vi "AutoTask Controller.vi"(8 "error in":errorcluster) -> ()   [LabVIEW 2015]
doc: "This VI executes continuously carrying out the current operation and responding to updates or new operations. It will often contain the timing or control code that is difficult to place directly in TeleOp. This VI generally opens all sensors and motors and isolates the rest of the robot code from knowing how the operations are carried out."
uses:
  AutoTask Setpoints.ctl
  AutoTask Operations.ctl
  <vilib>/Rock Robotics/Network Tables/NT Read Number.vi
  <vilib>/Rock Robotics/Network Tables/NT Write String.vi
  NavX/navX Library v2/navX Library v2.lvlib
  <vilib>/Rock Robotics/Network Tables/NT Write Boolean.vi
panel:
  out "Current\nCmd":string
  # "Tip: It may be helpful to observe inputs and sensor values.\nYou may also want to display tuning or debugging controls."
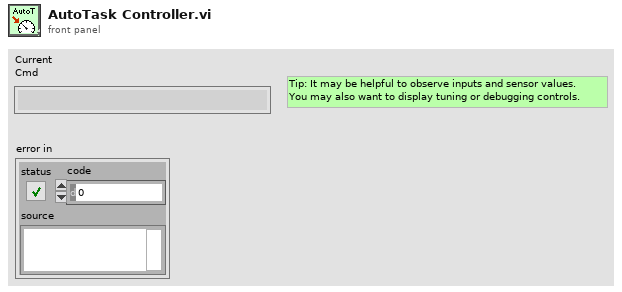
[diagram p1: front panel]
types:
  T1 = typedef "AutoTask Setpoints.ctl" = cluster{"Operation":T2, "Setpoint":dbl, "Duration":dbl, "Speed":dbl, "Angle":dbl, "VDeadband":dbl, "Deadband":dbl, "DriveSpeed":dbl}
  T2 = typedef "AutoTask Operations.ctl" = enum16{"Reserve", "Read Current", "Immediate", "DriveDistance", "AutoShoot", "FaceForward", "AutoAlign", "AutoTurn", "DriveToLine", "DriveToIncline", "DriveTillFlat"}
  T3 = typedef "navX Library v2.lvlib/Z900_navX_DeviceTypeDef.ctl" = cluster{"Interface":cluster{"Protocol":T4, "Update Rate (4Hz-60Hz)":u8, "navX Open TypeDef":variant}, "Notify Packet":refnum<notifier>, "Loop VI Refnum":refnum<vi>, "Ready to Close Occurrence Refnum":refnum<k4>}
  T4 = typedef "navX Library v2.lvlib/Z900_navX_ProtocolTypeDef.ctl" = enum16{"SERIAL", "I2C", "SPI"}
  T5 = typedef "Command Status Info.ctl" = cluster{"Name":string, "Status":T6, "notifier out":T7}
  T6 = typedef "Completion Status.ctl" = enum16{"Successful", "Aborted", "Incomplete"}
  T7 = typedef "Completion Notifier.ctl" = refnum<notifier>
  T8 = cluster{"Default Command":T1, "Command Timing":cluster{"Start Time (ms)":u32, "Iterations":i32}, "Command Arguments":cluster{"Command Info":T5, "Description":string, "Default Command":T1, "notifier out":refnum<notifier>, "Subsystem Name":string}}
  T9 = typedef "WPI_EncoderDevRef.ctl" = cluster{"DevStatus":errorcluster, "EncoderIndex":T10, "CounterIndex":T11, "DistancePerCount":dbl, "Decoding Type":T12}
  T10 = typedef "FPGA_EncoderIdx.ctl" = enum8{"Enc 0", "Enc 1", "Enc 2", "Enc 3", "Enc 4", "Enc 5", "Enc 6", "Enc 7", "Invalid"}
  T11 = typedef "FPGA_CounterCtrSystemIndex.ctl" = enum8{"Ctr 0", "Ctr 1", "Ctr 2", "Ctr 3", "Ctr 4", "Ctr 5", "Ctr 6", "Ctr 7", "Invalid"}
  T12 = typedef "WPI_EncoderType.ctl" = enum16{"1x", "2x", "4x"}
  T13 = cluster{"Yaw":dbl, "Roll":dbl, "Pitch":dbl, "Heading":dbl, "Fused Heading":dbl}
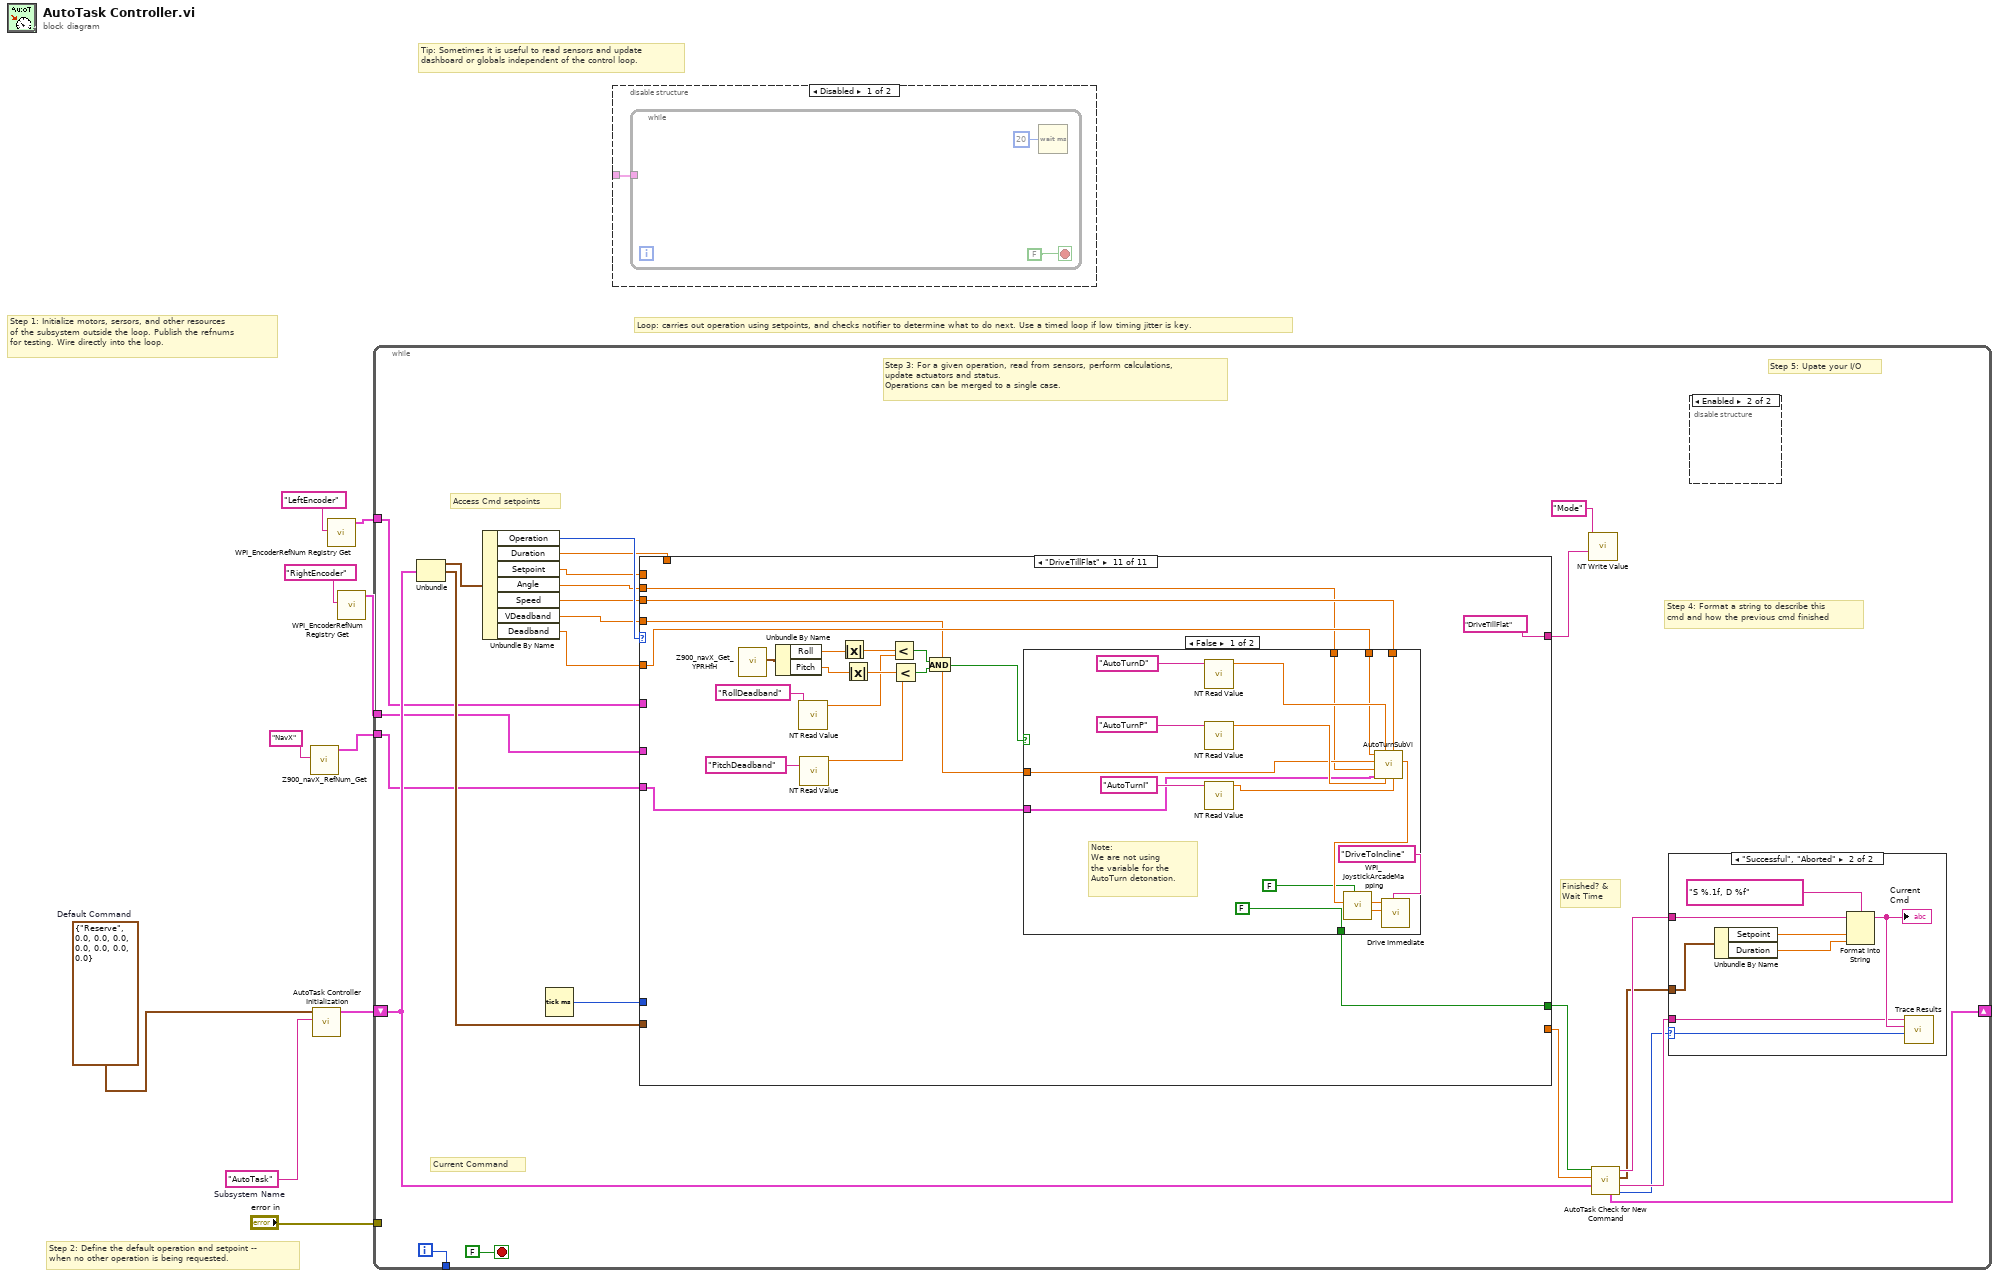
[diagram p0: block diagram]
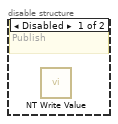
[diagram p3: hidden frame]
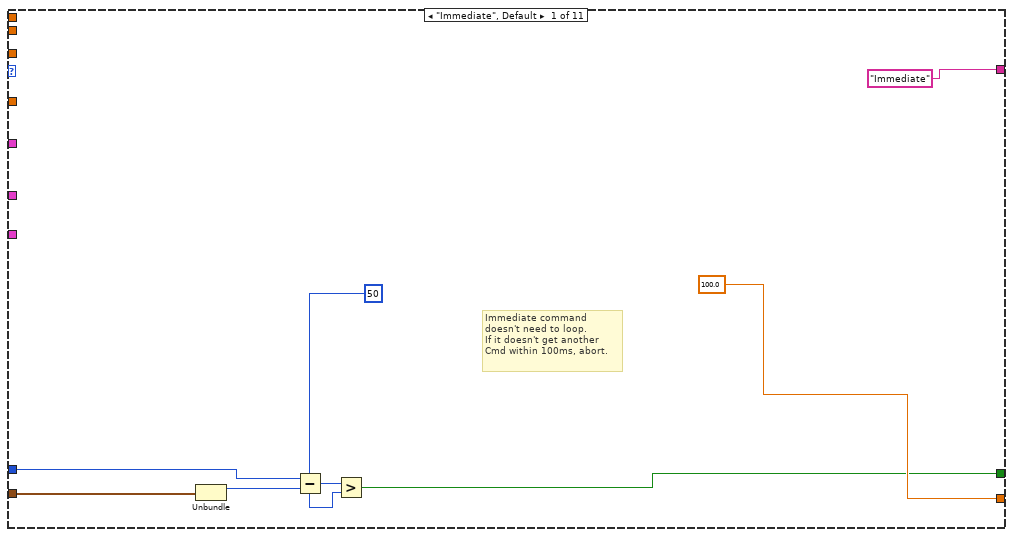
[diagram p5: hidden frame]
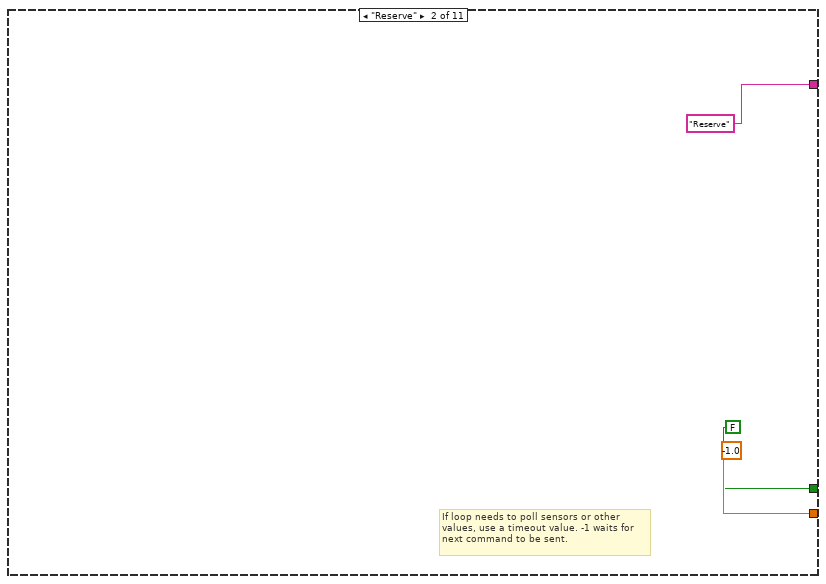
[diagram p6: hidden frame]
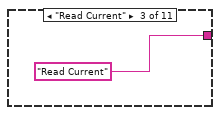
[diagram p7: hidden frame]
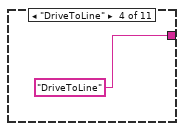
[diagram p8: hidden frame]
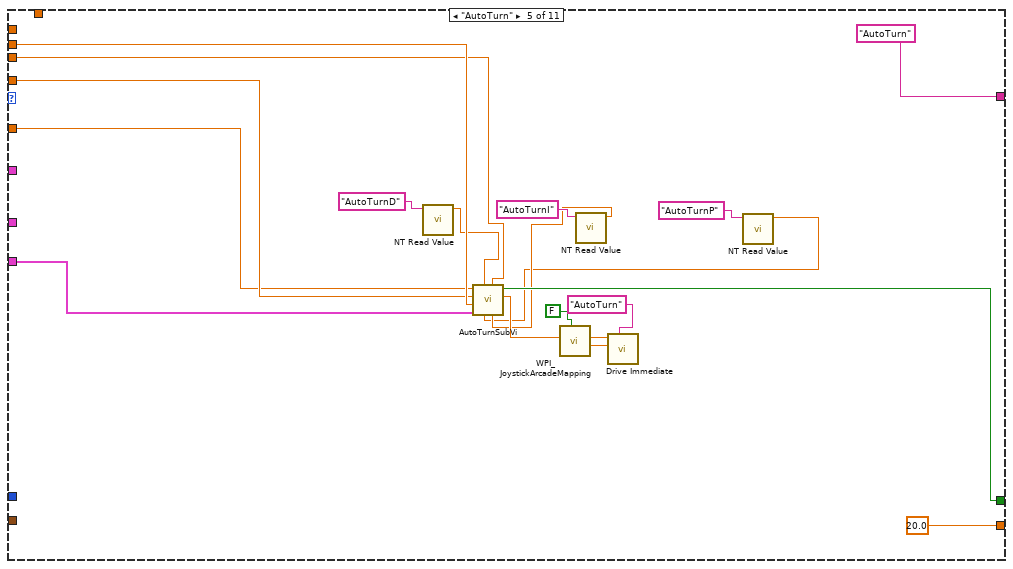
[diagram p9: hidden frame]
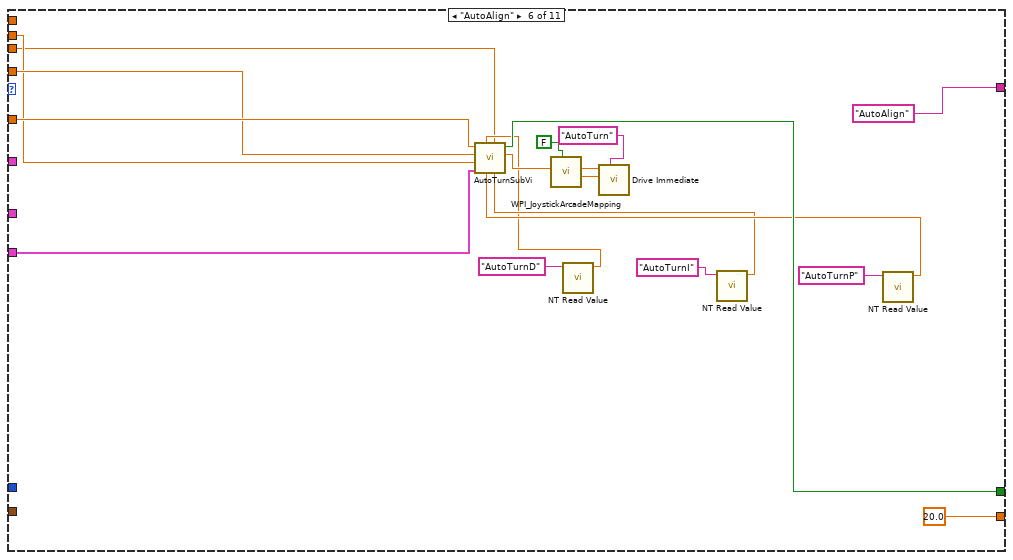
[diagram p10: hidden frame]
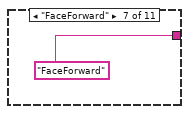
[diagram p11: hidden frame]
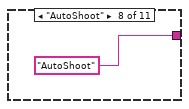
[diagram p12: hidden frame]
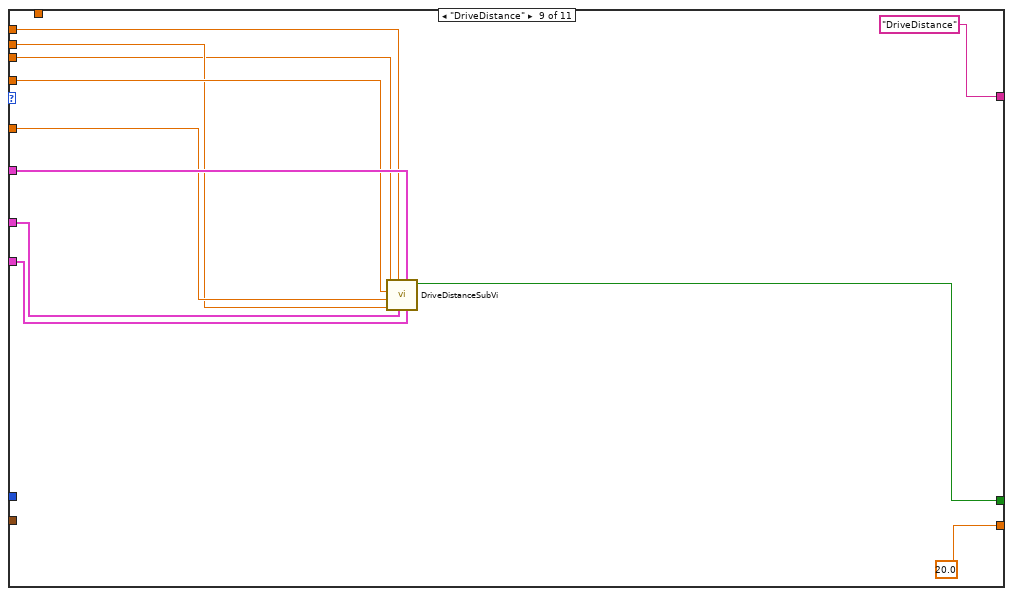
[diagram p13: hidden frame]
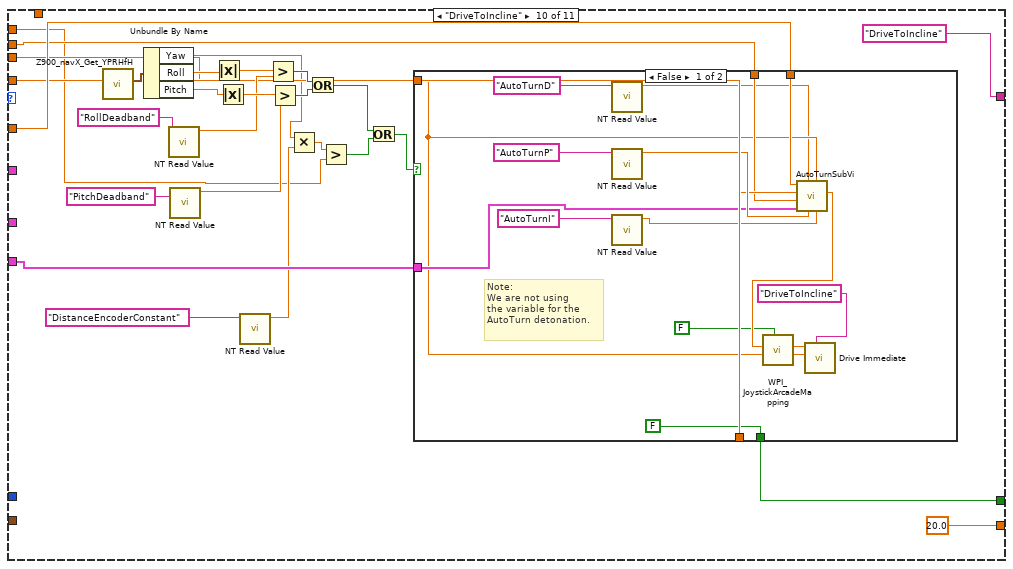
[diagram p14: hidden frame]
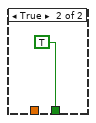
[diagram p15: hidden frame]
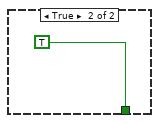
[diagram p16: hidden frame]
diagram:
  w7 = T1 {"Operation"=enum."Reserve", "Setpoint"=0.0, "Duration"=0.0, "Speed"=0.0, "Angle"=0.0, "VDeadband"=0.0, "Deadband"=0.0, "DriveSpeed"=0.0}  # Default Command
  w8 = "AutoTask"  # Subsystem Name
  # "Tip: Sometimes it is useful to read sensors and update\ndashboard or globals independent of the control loop."
  # "Step 2: Define the default operation and setpoint --\nwhen no other operation is being requested."
  # "Step 1: Initialize motors, sersors, and other resources\nof the subsystem outside the loop. Publish the refnums\nfor testing. Wire directly into the loop."
  # "Loop: carries out operation using setpoints, and checks notifier to determine what to do next. Use a timed loop if low timing jitter is key."
  n1 = call "Z900_navX_RefNum_Get.vi"("refnum name"="NavX") -> ("navX Device"=w6:T3)  [unwired: 9 in, 1 out]
  n2 = call "AutoTask Controller Initialization.vi"("Subsystem Name"=w8, "Default Command"=w7) -> ("Command Info"=w9:T8)  [unwired: 9 in]
  n3 = call <vilib>:"WPI_EncoderRefNum Registry Get.vi"("refnum name"="LeftEncoder") -> ("EncoderDevRef"=w2:T9)  [unwired: 9 in, 1 out]
  n4 = call <vilib>:"WPI_EncoderRefNum Registry Get.vi"("refnum name"="RightEncoder") -> ("EncoderDevRef"=w1:T9)  [unwired: 9 in, 1 out]
  n5 = while {
    shift-right: [w26] -> _
    shift-left: w9 -> [w27]
    tunnel: [w34] -> _
    tunnel: "error in" -> [_]
    tunnel: w6 -> [w19]
    tunnel: w2 -> [w15]
    tunnel: w1 -> [w14]
    i -> [w34]
    stop <- FALSE stop-if-true
    # "Step 5: Upate your I/O"
    # "Step 4: Format a string to describe this\ncmd and how the previous cmd finished"
    # "Current Command"
    # "Access Cmd setpoints"
    # "Finished? &\nWait Time"
    # "Step 3: For a given operation, read from sensors, perform calculations,\nupdate actuators and status.\nOperations can be merged to a single case."
    n6 = Unbundle(w27) -> ("Default Command"=w33:T1, "Command Timing"=w29:cluster{"Start Time (ms)":u32, "Iterations":i32})  [unwired: 1 out]
    n7 = Unbundle By Name(w33) -> ("Operation"=w32:T2, "Duration"=w31:dbl, "Setpoint"=w28:dbl, "Angle"=w18:dbl, "Speed"=w11:dbl, "VDeadband"=w13:dbl, "Deadband"=w12:dbl)
    n8 = Tick Count (ms)() -> (millisecond timer value=w30:u32)
    n9 = case shown="\"DriveTillFlat\"" w32 {
      tunnel: [100.0 -1.0 _ _ 20.0 20.0 _ _ 20.0 20.0 _] -> w24
      tunnel: [w45 FALSE ("ignore previous (F)") _ _ w71 w93 _ _ w98 w117 w160] -> w25
      tunnel: w29 -> [w47 _ _ _ _ _ _ _ _ _ _]
      tunnel: w31 -> [_ _ _ _ _ _ _ _ _ _ _]
      tunnel: w30 -> [w46 _ _ _ _ _ _ _ _ _ _]
      tunnel: w28 -> [_ _ _ _ _ _ _ _ w104 w111 _]
      tunnel: w19 -> [_ _ _ _ w73 w88 _ _ w97 w119 w154]
      tunnel: w18 -> [_ _ _ _ w74 w90 _ _ w101 w121 w155]
      tunnel: ["Immediate" "Reserve" "Read Current" "DriveToLine" "AutoTurn" "AutoAlign" "FaceForward" "AutoShoot" "DriveDistance" "DriveToIncline" "DriveTillFlat"] -> w16
      tunnel: w13 -> [_ _ _ _ w70 w91 _ _ w103 w122 w156]
      tunnel: w12 -> [_ _ _ _ w69 w92 _ _ w102 w123 w157]
      tunnel: w15 -> [_ _ _ _ _ _ _ _ w106 _ _]
      tunnel: w14 -> [_ _ _ _ _ _ _ _ w105 _ _]
      tunnel: w11 -> [_ _ _ _ w57 w76 _ _ w99 w120 w158]
      frame "Immediate", Default {
        # "Immediate command\ndoesn't need to loop.\nIf it doesn't get another\nCmd within 100ms, abort."
        n10 = Unbundle(w47) -> ("Start Time (ms)"=w50:u32)  [unwired: 1 out]
        n11 = Subtract(x=w46, y=w50) -> (x-y=w49:u32)
        n12 = Greater?(x=w49, y=u8 50 ("Left Motor")) -> (0:w45:bool)
      }
      frame "Reserve" {
        # "If loop needs to poll sensors or other\nvalues, use a timeout value. -1 waits for\nnext command to be sent."
      }
      frame "Read Current" {
      }
      frame "DriveToLine" {
      }
      frame "AutoTurn" {
        n13 = call-poly <vilib>:"NT Read Value.vi"("Name"="AutoTurnD") -> ("Numeric"=w59:dbl)  [unwired: 9 in, 1 out]
        n14 = call-poly <vilib>:"NT Read Value.vi"("Name"="AutoTurnI") -> ("Numeric"=w60:dbl)  [unwired: 9 in, 1 out]
        n15 = call-poly <vilib>:"NT Read Value.vi"("Name"="AutoTurnP") -> ("Numeric"=w58:dbl)  [unwired: 9 in, 1 out]
        n16 = call "AutoTurnSubVi.vi"("I"=w60, "Speed"=w57, "P"=w58, "D"=w59, "navX Device"=w73, "Angle"=w74, "VDeadband"=w70, "Deadband"=w69) -> ("Output"=w65:dbl, "Boolean"=w71:bool)  [unwired: 2 in]
        n17 = call <vilib>:"WPI_JoystickArcadeMapping.vi"("Square Inputs"=FALSE, "X axis value"=w65) -> ("Right Motor Value"=w67:dbl, "Left Motor Value"=w66:dbl)  [unwired: 8 in]
        n18 = call "Drive Immediate.vi"("Description"="AutoTurn", "Right Setpoint"=w67, "Left Setpoint"=w66) -> ()  [unwired: 8 in, 1 out]
      }
      frame "AutoAlign" {
        n19 = call-poly <vilib>:"NT Read Value.vi"("Name"="AutoTurnD") -> ("Numeric"=w77:dbl)  [unwired: 9 in, 1 out]
        n20 = call-poly <vilib>:"NT Read Value.vi"("Name"="AutoTurnI") -> ("Numeric"=w78:dbl)  [unwired: 9 in, 1 out]
        n21 = call-poly <vilib>:"NT Read Value.vi"("Name"="AutoTurnP") -> ("Numeric"=w79:dbl)  [unwired: 9 in, 1 out]
        n22 = call "AutoTurnSubVi.vi"("I"=w78, "Speed"=w76, "P"=w79, "D"=w77, "navX Device"=w88, "Angle"=w90, "VDeadband"=w91, "Deadband"=w92) -> ("Output"=w83:dbl, "Boolean"=w93:bool)  [unwired: 2 in]
        n23 = call <vilib>:"WPI_JoystickArcadeMapping.vi"("Square Inputs"=FALSE, "X axis value"=w83) -> ("Right Motor Value"=w86:dbl, "Left Motor Value"=w85:dbl)  [unwired: 8 in]
        n24 = call "Drive Immediate.vi"("Description"="AutoTurn", "Right Setpoint"=w86, "Left Setpoint"=w85) -> ()  [unwired: 8 in, 1 out]
      }
      frame "FaceForward" {
      }
      frame "AutoShoot" {
      }
      frame "DriveDistance" {
        n25 = call "DriveDistanceSubVi.vi"("navX Device"=w97, "EncoderDevRefLeft"=w106, "EncoderDevRefRight"=w105, "Setpoint"=w104, "Angle"=w101, "Deadband"=w102, "VDeadband"=w103, "Speed"=w99) -> ("Boolean"=w98:bool)  [unwired: 3 in]
      }
      frame "DriveToIncline" {
        n26 = call "Z900_navX_Get_YPRHfH.vi"() -> ("YRPHfH"=w134:T13)  [unwired: 8 in, 3 out]
        n27 = Unbundle By Name(w134) -> ("Yaw"=w115:dbl, "Roll"=w133:dbl, "Pitch"=w130:dbl)
        n28 = call-poly <vilib>:"NT Read Value.vi"("Name"="RollDeadband") -> ("Numeric"=w127:dbl)  [unwired: 9 in, 1 out]
        n29 = call-poly <vilib>:"NT Read Value.vi"("Name"="PitchDeadband") -> ("Numeric"=w126:dbl)  [unwired: 9 in, 1 out]
        n30 = Absolute Value(x=w133) -> (abs(x)=w132:dbl)
        n31 = Absolute Value(x=w130) -> (abs(x)=w131:dbl)
        n32 = call-poly <vilib>:"NT Read Value.vi"("Name"="DistanceEncoderConstant") -> ("Numeric"=w113:dbl)  [unwired: 9 in, 1 out]
        n33 = Greater?(x=w132, y=w127) -> (0:w124:bool)
        n34 = Greater?(x=w131, y=w126) -> (0:w125:bool)
        n35 = Multiply(x=w115, y=w113) -> (x*y=w112:dbl)
        n36 = Or(x=w124, y=w125) -> (x .or. y?=w110:bool)
        n37 = Greater?(x=w112, y=w111) -> (0:w109:bool)
        n38 = Or(x=w110, y=w109) -> (x .or. y?=w108:bool)
        n39 = case shown="False" w108 {
          tunnel: w123 -> [w141 _]
          tunnel: w122 -> [w140 _]
          tunnel: w121 -> [w139 _]
          tunnel: w120 -> [w137 _]
          tunnel: w119 -> [w138 _]
          tunnel: [FALSE TRUE] -> w117
          frame False {
            # "Note:\nWe are not using\nthe variable for the\nAutoTurn detonation."
            n40 = call-poly <vilib>:"NT Read Value.vi"("Name"="AutoTurnD") -> ("Numeric"=w135:dbl)  [unwired: 9 in, 1 out]
            n41 = call-poly <vilib>:"NT Read Value.vi"("Name"="AutoTurnP") -> ("Numeric"=w150:dbl)  [unwired: 9 in, 1 out]
            n42 = call-poly <vilib>:"NT Read Value.vi"("Name"="AutoTurnI") -> ("Numeric"=w149:dbl)  [unwired: 9 in, 1 out]
            n43 = call "AutoTurnSubVi.vi"("I"=w149, "Speed"=w137, "P"=w150, "D"=w135, "navX Device"=w138, "Angle"=w139, "VDeadband"=w140, "Deadband"=w141) -> ("Output"=w151:dbl)  [unwired: 2 in, 1 out]
            n44 = call <vilib>:"WPI_JoystickArcadeMapping.vi"("Square Inputs"=FALSE, "Y axis value"=w137, "X axis value"=w151) -> ("Right Motor Value"=w143:dbl, "Left Motor Value"=w142:dbl)  [unwired: 7 in]
            n45 = call "Drive Immediate.vi"("Description"="DriveToIncline", "Right Setpoint"=w143, "Left Setpoint"=w142) -> ()  [unwired: 8 in, 1 out]
          }
          frame True {
          }
        }
      }
      frame "DriveTillFlat" {
        n46 = call "Z900_navX_Get_YPRHfH.vi"() -> ("YRPHfH"=w171:T13)  [unwired: 8 in, 3 out]
        n47 = Unbundle By Name(w171) -> ("Roll"=w170:dbl, "Pitch"=w167:dbl)
        n48 = call-poly <vilib>:"NT Read Value.vi"("Name"="RollDeadband") -> ("Numeric"=w164:dbl)  [unwired: 9 in, 1 out]
        n49 = call-poly <vilib>:"NT Read Value.vi"("Name"="PitchDeadband") -> ("Numeric"=w163:dbl)  [unwired: 9 in, 1 out]
        n50 = Absolute Value(x=w170) -> (abs(x)=w169:dbl)
        n51 = Absolute Value(x=w167) -> (abs(x)=w168:dbl)
        n52 = Less?(x=w169, y=w164) -> (x < y?=w161:bool)
        n53 = Less?(x=w168, y=w163) -> (x < y?=w162:bool)
        n54 = And(x=w161, y=w162) -> (x .and. y?=w159:bool)
        n55 = case shown="False" w159 {
          tunnel: [FALSE TRUE] -> w160
          tunnel: w158 -> [w177 _]
          tunnel: w157 -> [w176 _]
          tunnel: w156 -> [w175 _]
          tunnel: w155 -> [w174 _]
          tunnel: w154 -> [w172 _]
          frame False {
            # "Note:\nWe are not using\nthe variable for the\nAutoTurn detonation."
            n56 = call-poly <vilib>:"NT Read Value.vi"("Name"="AutoTurnD") -> ("Numeric"=w178:dbl)  [unwired: 9 in, 1 out]
            n57 = call-poly <vilib>:"NT Read Value.vi"("Name"="AutoTurnP") -> ("Numeric"=w187:dbl)  [unwired: 9 in, 1 out]
            n58 = call-poly <vilib>:"NT Read Value.vi"("Name"="AutoTurnI") -> ("Numeric"=w173:dbl)  [unwired: 9 in, 1 out]
            n59 = call "AutoTurnSubVi.vi"("I"=w173, "Speed"=w177, "P"=w187, "D"=w178, "navX Device"=w172, "Angle"=w174, "VDeadband"=w175, "Deadband"=w176) -> ("Output"=w188:dbl)  [unwired: 2 in, 1 out]
            n60 = call <vilib>:"WPI_JoystickArcadeMapping.vi"("Square Inputs"=FALSE, "X axis value"=w188) -> ("Right Motor Value"=w181:dbl, "Left Motor Value"=w180:dbl)  [unwired: 8 in]
            n61 = call "Drive Immediate.vi"("Description"="DriveToIncline", "Right Setpoint"=w181, "Left Setpoint"=w180) -> ()  [unwired: 8 in, 1 out]
          }
          frame True {
          }
        }
      }
    }
    n62 = call-poly <vilib>:"NT Write Value.vi"("String"=w16, "Name"="Mode") -> ()  [unwired: 9 in, 1 out]
    n63 = call "AutoTask Check for New Command.vi"("Current Command"=w27, "Wait time (ms)"=w24, "Finished?"=w25) -> ("Completion"=w20:T6, "Subsystem Name"=w21:string, "Current Command"=w22:T1, "Initial Trace String"=w23:string, "NextCommand"=w26:T8)  [unwired: 4 in]
    n64 = case shown="\"Successful\", \"Aborted\"" w20 {
      selector: w20 -> [_ w43]
      tunnel: w23 -> [_ w39]
      tunnel: w22 -> [_ w40]
      tunnel: w21 -> [_ w36]
      frame "Incomplete", Default {
        # "Continuing current command"
      }
      frame "Successful", "Aborted" {
        # "Report and setup for next command"
        n65 = Unbundle By Name(w40) -> ("Setpoint"=w42:dbl, "Duration"=w37:dbl)
        n66 = Format Into String(format string="S %.1f, D %f", initial string=w39, w42, w37) -> (resulting string=w38:string)  [unwired: 1 in, 1 out]
        "Current\nCmd" <- w38
        n67 = call <vilib>:"Trace Results.vi"("Status of previous command"=w43, "Description"=w38, "Subsystem"=w36) -> ()  [unwired: 9 in]
      }
    }
    n68 = disable-structure shown="Enabled" {
      frame Disabled {
        # "Publish"
        n69 = call-poly <vilib>:"NT Write Value.vi"() -> ()  [unwired: 11 in, 1 out]
      }
      frame Enabled {
      }
    }
  }
  n70 = disable-structure shown="Disabled" {
    disable-tunnel: _ -> [w190 _]
    frame Disabled {
      n71 = while {
        tunnel: w190 -> [_]
        stop <- FALSE stop-if-true
        n72 = Wait (ms)(milliseconds to wait=u32 20) -> ()  [unwired: 1 out]
      }
    }
    frame Enabled {
    }
  }
